vi "SetDisplayDigits.vi"(8 "Error In":errorcluster, 10 "Resolution (Number of Digits)":u8=6 min=4 max=7 step=1, 11 "Keithley 6482 In":refnum<visa-resource-name>) -> (0 "Error Out":errorcluster, 3 "Keithley 6482 Out":refnum<visa-resource-name>)   [LabVIEW 2014, in "Keithley-6482-Visa.lvlib"]
uses:
  Keithley-6482-Visa.lvlib
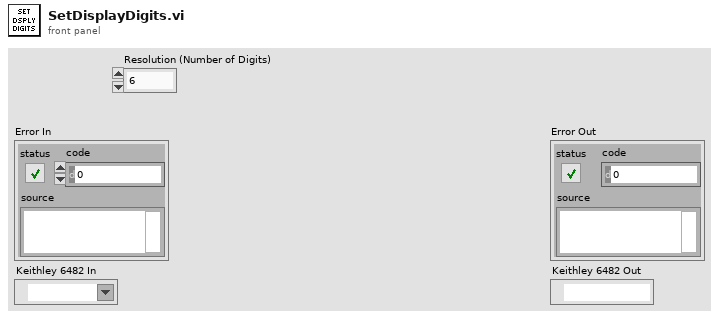
[diagram p1: front panel]
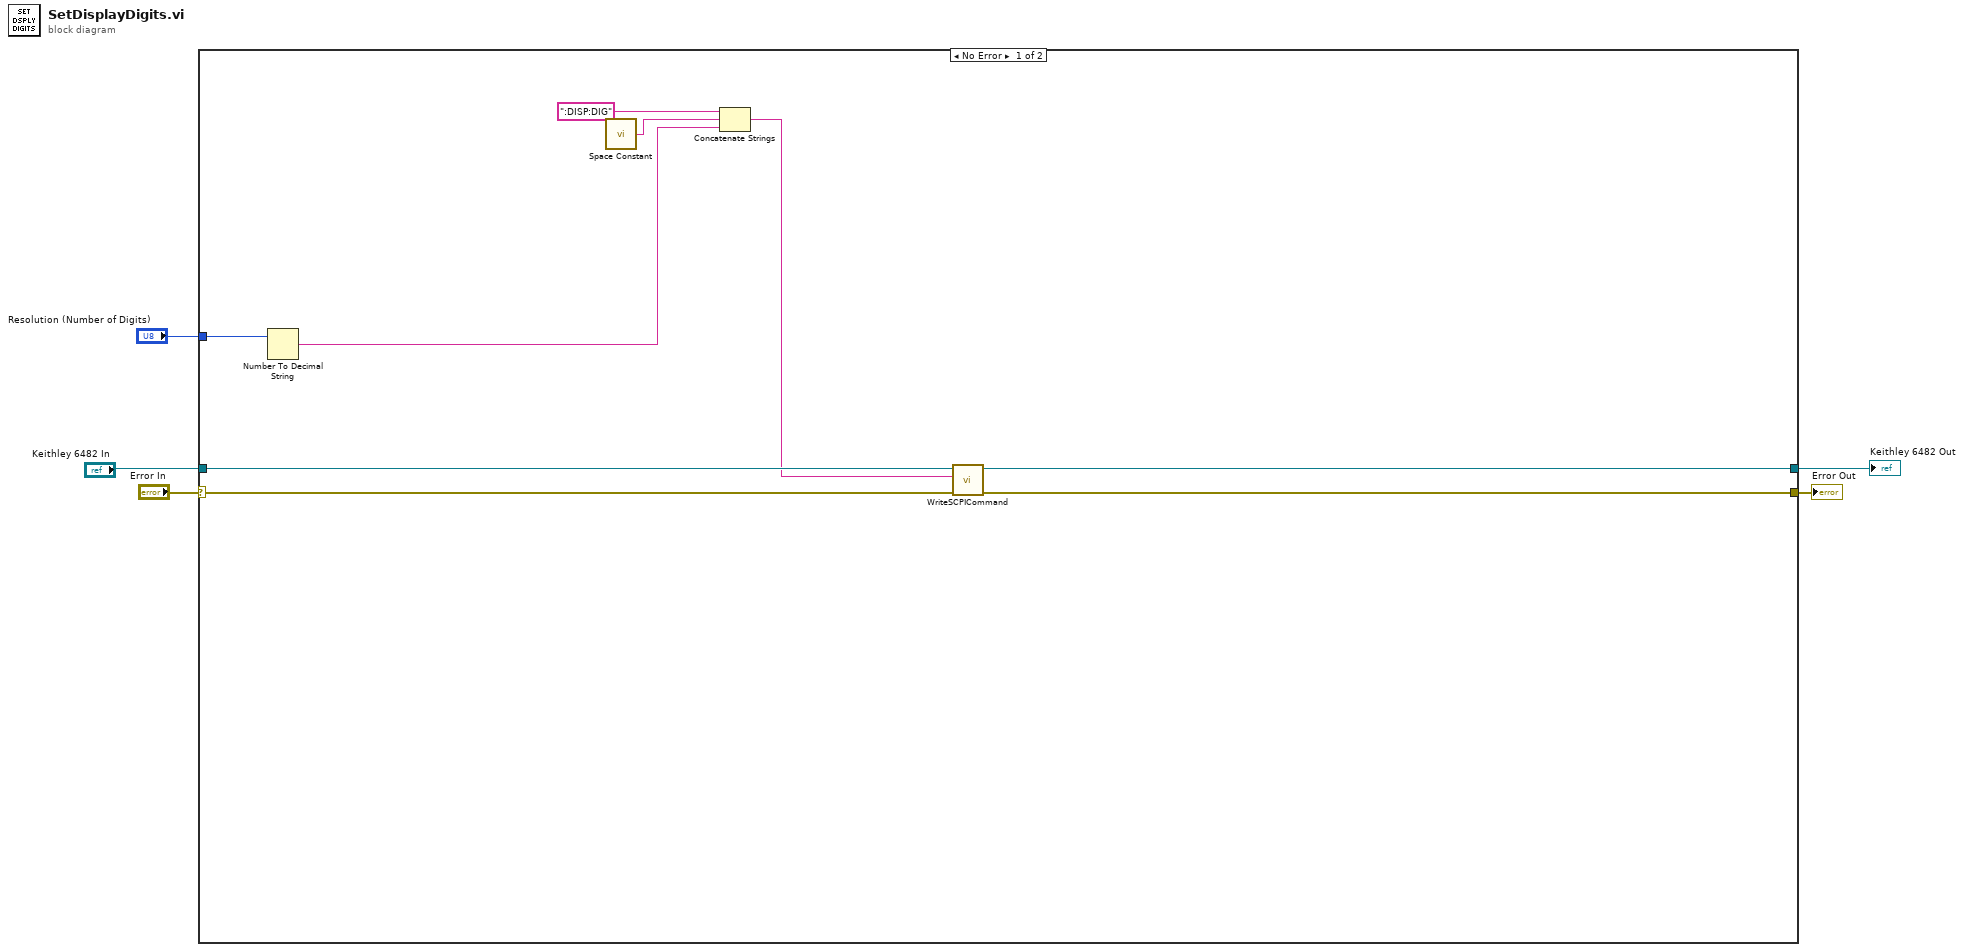
[diagram p0: block diagram]
diagram:
  n1 = case shown="No Error" "Error In" {
    selector: "Error In" -> [w9 w15]
    tunnel: [w8 w15] -> w4
    tunnel: [w7 w16] -> w3
    tunnel: "Keithley 6482 In" -> [w10 w16]
    tunnel: "Resolution (Number of Digits)" -> [w12 _]
    frame No Error {
      n2 = Number To Decimal String(number=w12) -> (decimal integer string=w11:string)  [unwired: 1 in]
      n3 = call <vilib>:"Space Constant.vi"() -> ("String"=w13:string)
      n4 = Concatenate Strings(":DISP:DIG", w13, w11) -> (w6:string)
      n5 = call "WriteSCPICommand.vi"("Error In"=w9, "SCPI Command"=w6, "Keithley 6482 In"=w10) -> ("Error Out"=w8:errorcluster, "Keithley 6482 Out"=w7:refnum<visa-resource-name>)  [unwired: 7 in]
    }
    frame Error {
    }
  }
  "Error Out" <- w4
  "Keithley 6482 Out" <- w3
